vi "CRYDataView Virtual Window.vi"   [LabVIEW 2013]
uses:
  SubVI/CRYMain Sub Window Global.vi
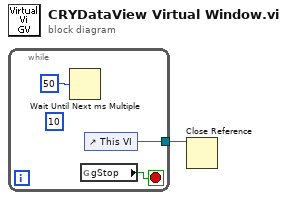
[diagram p0: block diagram]
diagram:
  n1 = while {
    tunnel: [w3] -> w1
    stop <- w2 stop-if-true
    (unwired) 10
    n2 = Wait Until Next ms Multiple(millisecond multiple=u32 50) -> ()  [unwired: 1 out]
    n3 = global read "CRYMain Sub Window Global.vi" "gStop"() -> (w2:bool)
    n4 = control-ref of="This VI"() -> (w3:refnum<vi>)
  }
  n5 = Close Reference(reference=w1) -> ()  [unwired: 1 in, 1 out]
